vi "FPGA_WaitOnInterrupt.vi"(8 "error in (no error)":errorcluster, 9 "Ignore Previous Interrupts":bool, 10 "Timeout (ms)":i32=-1, 11 "InteruptRef":T1) -> (0 "error out":errorcluster, 1 "IRQ Asserted":i32, 2 "Timed Out":bool, 3 "InteruptRef":T1)   [LabVIEW 2017]
uses:
  <vilib>/Rock Robotics/SystemInterfaces/Interrupt/FPGA_InterruptRef.ctl
  <vilib>/Rock Robotics/SystemInterfaces/Interrupt/FPGA_InterruptIndex.ctl
  <vilib>/Utility/error.llb/Error Cluster From Error Code.vi
  <vilib>/rvi/errors/niLvFpgaAdjustHostInterfaceError.vi
  <vilib>/RVI Host/nirviSupport.llb/nirviErrorClusterFromErrorCode.vi
  <vilib>/Rock Robotics/SystemInterfaces/System/FPGA_SystemFPGA Ref Global.vi
  <vilib>/Rock Robotics/SystemInterfaces/System/FPGA_SystemFRC FPGA Ref.ctl
  <vilib>/rvi/interface/nirviMethod/nirviMethod.xnode
  <vilib>/FPGAPlugInAG/Dynamic/niLvFpga_AcknowledgeIrq_Dynamic.vi
  <vilib>/rvi/interface/nirviMethod/StockFPGA_InlinedMethodWaitForSingleIRQ.vi
  <vilib>/FPGAPlugInAG/Dynamic/niLvFpga_WaitOnIrq_Dynamic.vi
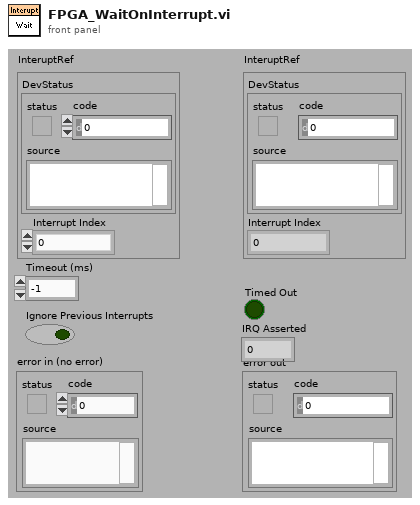
[diagram p1: front panel]
types:
  T1 = typedef "FPGA_InterruptRef.ctl" = cluster{"DevStatus":errorcluster, "Interrupt Index":T2}
  T2 = typedef "FPGA_InterruptIndex.ctl" = enum8{"0", "1", "2", "3", "4", "5", "6", "7", "Invalid"}
  T3 = typedef "FPGA_SystemFRC FPGA Ref.ctl" = refnum<k20>
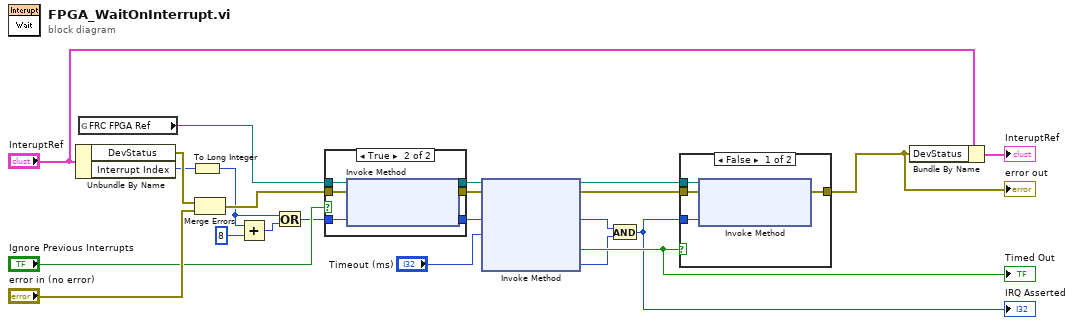
[diagram p0: block diagram]
diagram:
  n1 = Unbundle By Name("InteruptRef") -> ("DevStatus"=w10:errorcluster, "Interrupt Index"=w6:T2)
  n2 = global read "FPGA_SystemFPGA Ref Global.vi" "FRC FPGA Ref"() -> (w18:T3)
  n3 = To Long Integer(number=w6) -> (32bit integer=w5:i32)
  n4 = Merge Errors(w10, "error in (no error)") -> (w11:errorcluster)
  n5 = Add(x=w5, y=8) -> (x+y=w2:i32)
  n6 = Or(x=w5, y=w2) -> (x .or. y?=w3:i32)
  n7 = case shown="True" "Ignore Previous Interrupts" {
    tunnel: w18 -> [w25 w30]
    tunnel: [w25 w29] -> w14
    tunnel: [w24 w28] -> w13
    tunnel: w3 -> [w23 w26]
    tunnel: w11 -> [w24 w27]
    tunnel: [w23 w26] -> w8
    frame False {
    }
    frame True {
      n8 = xnode "Invoke Method"("FPGA VI Reference In"=w30, "error in"=w27, "IRQ Number(s)"=w26) -> ("FPGA VI Reference Out"=w29:T3, "error out"=w28:errorcluster)
    }
  }
  n9 = xnode "Invoke Method"("FPGA VI Reference In"=w14, "error in"=w13, "IRQ Number(s)"=w8, "Timeout (ms)"="Timeout (ms)") -> ("FPGA VI Reference Out"=w15:T3, "error out"=w17:errorcluster, "Timed Out"=w19:bool, "IRQ(s) Asserted"=w7:i32)
  "Timed Out" <- w19
  n10 = And(x=w8, y=w7) -> (x .and. y?=w1:i32)
  "IRQ Asserted" <- w1
  n11 = case shown="False" w19 {
    tunnel: w17 -> [w34 w35]
    tunnel: [w33 w35] -> w20
    tunnel: w15 -> [w32 _]
    tunnel: w1 -> [w31 _]
    frame False {
      n12 = xnode "Invoke Method"("FPGA VI Reference In"=w32, "error in"=w34, "IRQ Number(s)"=w31) -> ("error out"=w33:errorcluster)  [unwired: 1 out]
    }
    frame True {
    }
  }
  "error out" <- w20
  n13 = Bundle By Name(cluster="InteruptRef", "DevStatus"=w20) -> (→"InteruptRef":T1)
